vi "compute cluster centers double.vi"(0 "dataset":dbl[][](array[numeric]), 1 "clusters":i32, 3 "Overwrite Lib Path":path, 9 "flann_params":T1={"algorithm"=4, "checks"=32, "eps"=0.0, "sorted"=1, "max_neighbors"=-1, "cores"=0, "trees"=1, "leaf_max_size"=4, "branching"=32, "iterations"=5, "centers_init"=0, "cb_index"=0.5, "target_precision"=0.9, "build_weight"=0.01, "memory_weight"=0.0, "sample_fraction"=0.1, "table_number_"=12, "key_size_"=20, "multi_probe_level_"=2, "log_level"=0, "random_seed"=-1} {"algorithm" items=["FLANN_INDEX_LINEAR"=0, "FLANN_INDEX_KDTREE"=1, "FLANN_INDEX_KMEANS"=2, "FLANN_INDEX_COMPOSITE"=3, "FLANN_INDEX_KDTREE_SINGLE"=4, "FLANN_INDEX_HIERARCHICAL"=5, "FLANN_INDEX_LSH"=6, "FLANN_INDEX_SAVED"=254, "FLANN_INDEX_AUTOTUNED"=255]; "centers_init" items=["FLANN_CENTERS_RANDOM", "FLANN_CENTERS_GONZALES", "FLANN_CENTERS_KMEANSPP", "FLANN_CENTERS_GROUPWISE"]; "log_level" items=["FLANN_LOG_NONE", "FLANN_LOG_FATAL", "FLANN_LOG_ERROR", "FLANN_LOG_WARN", "FLANN_LOG_INFO", "FLANN_LOG_DEBUG"]}, 11 "error in (no error)":errorcluster) -> (4 "result out":dbl[][](array[numeric]), 10 "flann_params":T1 {"algorithm" items=["FLANN_INDEX_LINEAR"=0, "FLANN_INDEX_KDTREE"=1, "FLANN_INDEX_KMEANS"=2, "FLANN_INDEX_COMPOSITE"=3, "FLANN_INDEX_KDTREE_SINGLE"=4, "FLANN_INDEX_HIERARCHICAL"=5, "FLANN_INDEX_LSH"=6, "FLANN_INDEX_SAVED"=254, "FLANN_INDEX_AUTOTUNED"=255]; "centers_init" items=["FLANN_CENTERS_RANDOM", "FLANN_CENTERS_GONZALES", "FLANN_CENTERS_KMEANSPP", "FLANN_CENTERS_GROUPWISE"]; "log_level" items=["FLANN_LOG_NONE", "FLANN_LOG_FATAL", "FLANN_LOG_ERROR", "FLANN_LOG_WARN", "FLANN_LOG_INFO", "FLANN_LOG_DEBUG"]}, 15 "error out":errorcluster)   [LabVIEW 2020, in "KD Tree.lvlib"]
doc: "FLANN_EXPORT int flann_compute_cluster_centers_double(double* dataset,\n int rows,\n int cols,\n int clusters,\n double* result,\n struct FLANNParameters* flann_params);"
uses:
  KD Tree.lvlib
  Flann Params.ctl
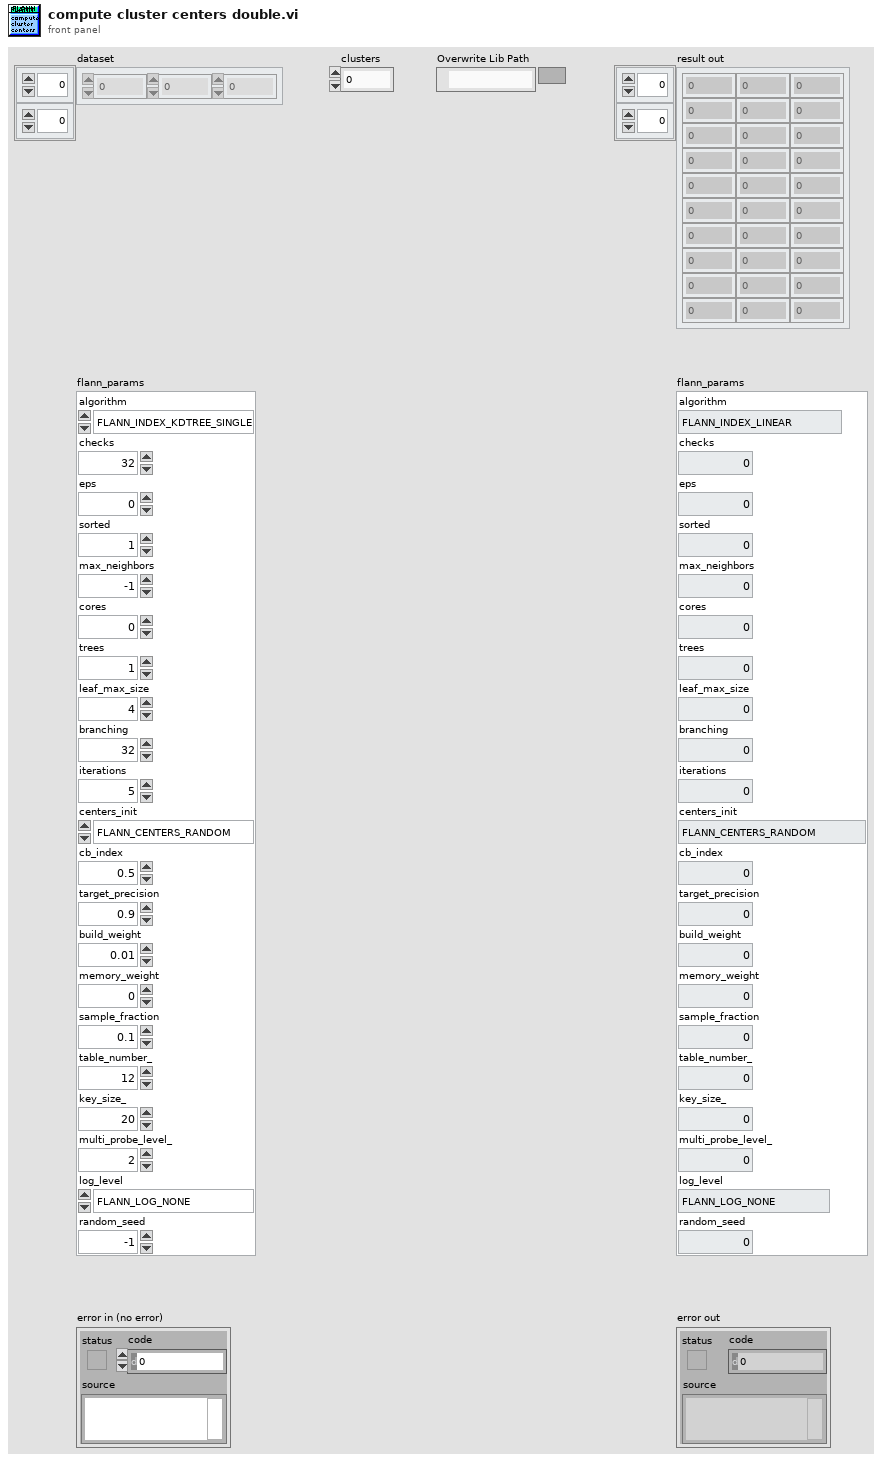
[diagram p1: front panel]
types:
  T1 = typedef "KD Tree.lvlib/Flann Params.ctl" = cluster{"algorithm":u32, "checks":i32, "eps":sgl, "sorted":i32, "max_neighbors":i32, "cores":i32, "trees":i32, "leaf_max_size":i32, "branching":i32, "iterations":i32, "centers_init":u32, "cb_index":sgl, "target_precision":sgl, "build_weight":sgl, "memory_weight":sgl, "sample_fraction":sgl, "table_number_":u32, "key_size_":u32, "multi_probe_level_":u32, "log_level":u32, "random_seed":i32}
  T2 = typedef "Semaphore RefNum" = refnum<k1>
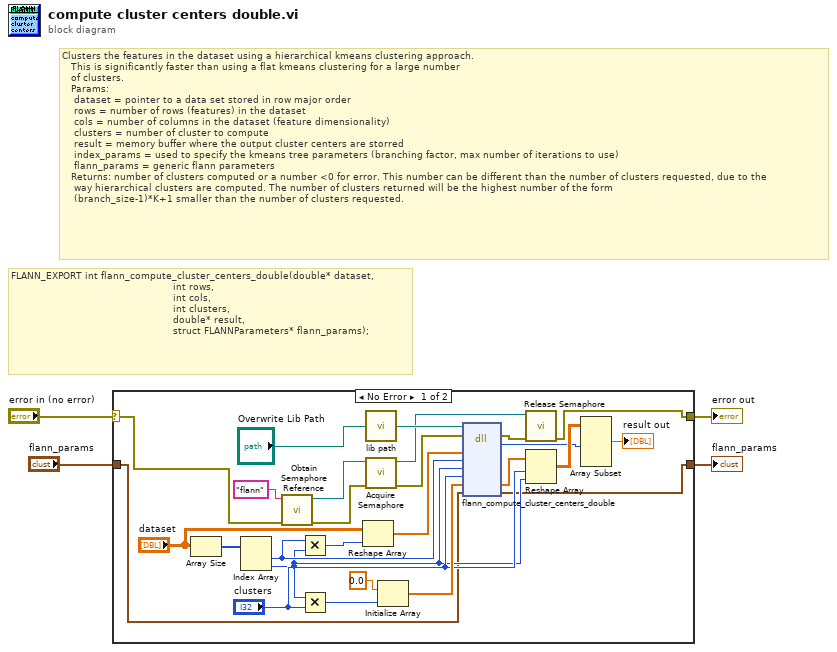
[diagram p0: block diagram]
diagram:
  # "Clusters the features in the dataset using a hierarchical kmeans clustering approach.\n   This is significantly faster than using a flat kmeans clustering for a large number\n   of clusters.\n   Params:\n    dataset = pointer to a data set stored in row major order\n    rows = number of rows (features) in the dataset\n    cols = number of columns in the dataset (feature dimensionality)\n    clusters = number of cluster to compute\n    result = memory buffer where the output cluster centers are storred\n    index_params = used to specify the kmeans tree parameters (branching factor, max number of iterations to use)\n    flann_params = generic flann parameters\n   Returns: number of clusters computed or a number <0 for error. This number can be different than the number of clusters requested, due to the\n    way hierarchical clusters are computed. The number of clusters returned will be the highest number of the form\n    (branch_size-1)*K+1 smaller than the number of clusters requested."
  # "FLANN_EXPORT int flann_compute_cluster_centers_double(double* dataset,\n                                                      int rows,\n                                                      int cols,\n                                                      int clusters,\n                                                      double* result,\n                                                      struct FLANNParameters* flann_params);"
  n1 = case shown="No Error" "error in (no error)" {
    selector: "error in (no error)" -> [w18 w32]
    tunnel: [w6 w32] -> w3
    tunnel: "flann_params" -> [w15 w31]
    tunnel: [w14 w31] -> w1
    frame No Error {
      n2 = Array Size(array="dataset") -> (size(s)=w28:i32[])
      n3 = Index Array(array=w28) -> (element #1=w26:i32, element #2=w21:i32)  [unwired: 2 in]
      n4 = call <vilib>:"Obtain Semaphore Reference.vi"("error in (no error)"=w18, "name (unnamed)"="flann") -> ("error out"=w10:errorcluster, "semaphore"=w7:T2)  [unwired: 3 in, 1 out]
      n5 = Multiply(x=w26, y=w21) -> (x*y=w27:i32)
      n6 = Multiply(x=w21, y="clusters") -> (x*y=w24:i32)
      n7 = Reshape Array("dataset", w27) -> (w29:dbl[])
      n8 = call "lib path.vi"("Overwrite Lib Path"="Overwrite Lib Path") -> ("lib path"=w12:path)
      n9 = call <vilib>:"Acquire Semaphore.vi"("error in (no error)"=w10, "semaphore"=w7) -> ("error out"=w8:errorcluster, "semaphore out"=w5:T2)  [unwired: 3 in, 1 out]
      n10 = Initialize Array(0.0, w24) -> (w25:dbl[])
      n11 = dll-call lib="E:/Labview/LV 2020/Libs/flann/flann.*" fn="flann_compute_cluster_centers_double"(path in=w12, error in=w8, "dataset"=w29, "rows"=w26, "cols"=w21, "clusters"="clusters", "result"=w25, "flann_params"=w15) -> (error out=w17:errorcluster, "return type"=w19:i32, "result"=w23:dbl[], "flann_params"=w14:T1)  [unwired: 5 in, 1 out]
      n12 = call <vilib>:"Release Semaphore.vi"("error in (no error)"=w17, "semaphore"=w5) -> ("error out"=w6:errorcluster)  [unwired: 4 in, 1 out]
      n13 = Reshape Array(w23, "clusters", w21) -> (w20:dbl[][])
      n14 = Array Subset(array=w20, length (row)=w19) -> (→"result out":dbl[][])  [unwired: 3 in]
    }
    frame Error {
    }
  }
  "error out" <- w3
  "flann_params" <- w1
